vi "ConfigParams - Parse - UDPData.vi"(8 "error in (no error)":errorcluster, 11 "Ethernet in":refnum<class "ENET_BS1201.lvclass">) -> (0 "error out":errorcluster, 1 "UDPDataPeriod_mS":i32=5, 2 "UDP Data Port":i32=54321, 3 "Ethernet out":refnum<class "ENET_BS1201.lvclass">, 5 "UDP Data Enable":bool=TRUE)   [LabVIEW 2021, in "BS120x Driver.lvlib" / "ENET_BS1201.lvclass"]
uses:
  ENET_BS1201.lvclass
panel:
  # "[UDPData]\nUDPDataEnable = True\nUDPDataPort = 54322\nUDPDataPeriod_mS = 5"
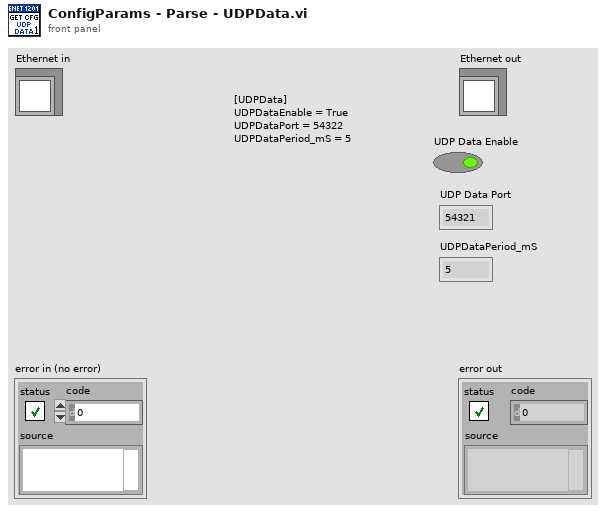
[diagram p1: front panel]
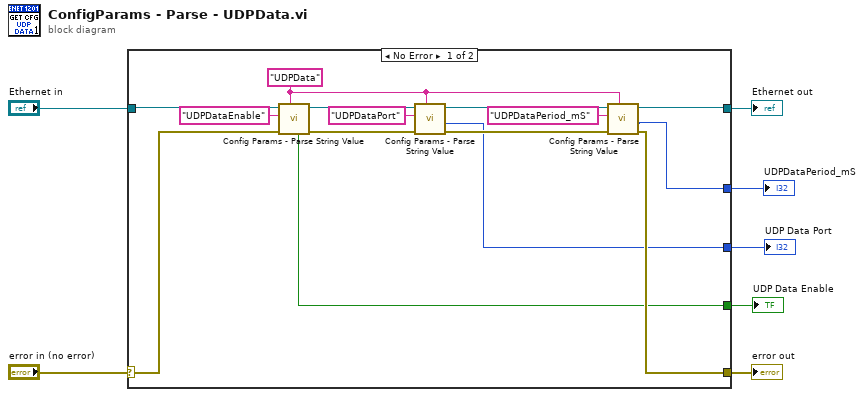
[diagram p0: block diagram]
diagram:
  n1 = case shown="No Error" "error in (no error)" {
    selector: "error in (no error)" -> [w13 w24]
    tunnel: [w11 w24] -> w6
    tunnel: [w14 w23] -> w4
    tunnel: "Ethernet in" -> [w22 w23]
    tunnel: [w10 _] -> w3
    tunnel: [w9 _] -> w2
    tunnel: [w8 _] -> w1
    frame No Error {
      w16 = "UDPData" ("Section")
      n2 = call-dynamic "Config Params - Parse String Value.vi"("Section"=w16, "error in (no error)"=w13, "Key"="UDPDataEnable", "Ethernet in"=w22) -> ("error out"=w12:errorcluster, "Ethernet out"=w20:refnum<class "ENET_BS1201.lvclass">, "Value (bool)"=w10:bool)  [unwired: 1 in, 4 out]
      n3 = call-dynamic "Config Params - Parse String Value.vi"("Section"=w16, "error in (no error)"=w12, "Key"="UDPDataPort", "Ethernet in"=w20) -> ("error out"=w17:errorcluster, "Value (int)"=w9:i32, "Ethernet out"=w18:refnum<class "ENET_BS1201.lvclass">)  [unwired: 1 in, 4 out]
      n4 = call-dynamic "Config Params - Parse String Value.vi"("Section"=w16, "error in (no error)"=w17, "Key"="UDPDataPeriod_mS", "Ethernet in"=w18) -> ("error out"=w11:errorcluster, "Value (int)"=w8:i32, "Ethernet out"=w14:refnum<class "ENET_BS1201.lvclass">)  [unwired: 1 in, 4 out]
    }
    frame Error {
    }
  }
  "error out" <- w6
  "Ethernet out" <- w4
  "UDP Data Enable" <- w3
  "UDP Data Port" <- w2
  "UDPDataPeriod_mS" <- w1
